vi "VISA02_ModbusRTU01_Read.vi"(11 "YTESTER测试数据":T1={"Socket(From1)"=1, "SN"=refnum, "StopFlagRef"=refnum, "YT System Queue"=refnum}) -> (3 "YTESTER结论":T2)   [LabVIEW 2017]
doc: "VIDescription=基于NI官方库的MODBUS操作"
uses:
  YtCommon.lvlibp/yt`Step StepBaseInput.ctl
  YtCommon.lvlibp/yt`Step StepResult.ctl
  YtCommon.lvlibp/yt`Step TestData.ctl
  YtCommon.lvlibp/yt`Step System Queue.ctl
  Step`s VIs/YYLLGeneric/variable_W.ctl
  YtCommon.lvlibp/yt`Data-Ytester Type Data.ctl
  Step`s VIs/NI Modbus.llb/MB Serial Master Query Read Discrete Inputs (poly).vi
  Step`s VIs/NI Modbus.llb/MB Serial Master Query Read Coils (poly).vi
  Step`s VIs/NI Modbus.llb/MB Serial Master Query Read Input Registers (poly).vi
  Step`s VIs/NI Modbus.llb/MB Serial Master Query Read Holding Registers (poly).vi
  YtCommon.lvlibp
panel:
  out "Read Registers":u16[](array[numeric]) format="%.0x"
  out "Read Bits":bool[](array[boolean])
  in  "YTESTER开放参数":T4={"YTESTER_BaseInput"={"isTest"=FALSE, "isSkip"=FALSE, "StepName"="NI Modbus读", "OnPass"=enum."Next", "OnFail"=enum."Next", "ReTestNumber"=0.0}, "VISA resource"="", "baud rate (9600)"="9600", "Mode"=enum."RTU", "ReadType"=enum."Discretes Input", "Slave Address"=1, "Timeout"=3000, "Starting Address"=0, "Quantity"=1} {"Starting Address" format="%.0x"}
  # "Modbus\nRead"
  # "#yyll 采用NI-Modbus VI 内部存在耗时，待优化！！！"
  # "Modbus四种数据类型：\n　　Discretes Input　　　　     位变量            只读\n　　Coils　　　　　　　　    　 位变量            读写\n　　Input Registers　　   　16-bit整型            只读\n　　Holding Registers 　    16-bit整型            读写"
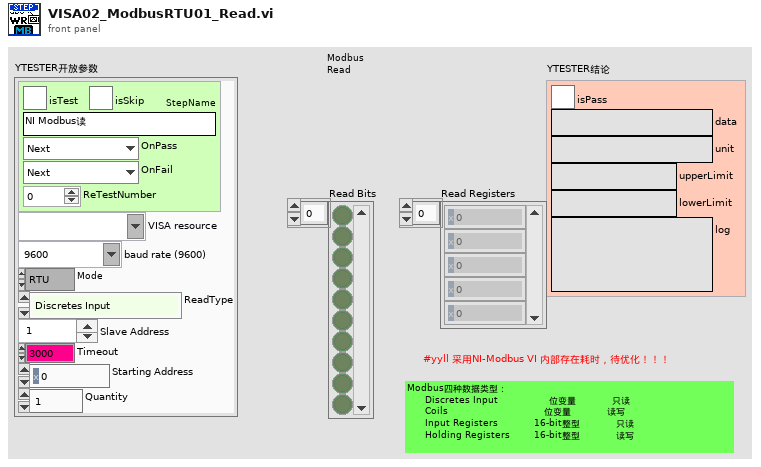
[diagram p1: front panel]
types:
  T1 = typedef "YtCommon.lvlibp/yt`Step TestData.ctl" = cluster{"Socket(From1)":i32, "SN":refnum<notifier>, "StopFlagRef":refnum<notifier>, "YT System Queue":refnum<queue>}
  T2 = typedef "YtCommon.lvlibp/yt`Step StepResult.ctl" = cluster{"isPass":bool, "data":string, "unit":string, "upperLimit":string, "lowerLimit":string, "log":string}
  T3 = typedef "YtCommon.lvlibp/yt`Step StepBaseInput.ctl" = cluster{"isTest":bool, "isSkip":bool, "StepName":string, "OnPass":enum16{"Next", "ToOVER", "Terminate"}, "OnFail":enum16{"Next", "ToOVER", "Terminate"}, "ReTestNumber":dbl}
  T4 = cluster{"YTESTER_BaseInput":T3, "VISA resource":refnum<visa-resource-name>, "baud rate (9600)":string, "Mode":enum16{"RTU", "ASCII"}, "ReadType":enum16{"Discretes Input", "Coils", "Input Registers", "Holding Registers"}, "Slave Address":u8, "Timeout":u32, "Starting Address":u16, "Quantity":u16}
  T5 = cluster{"Mode":enum16{"RTU", "ASCII"}, "Slave Address":u8}
  T6 = enum16{"Discretes Input", "Coils", "Input Registers", "Holding Registers"}
  T7 = typedef "variable_W.ctl" = cluster{"YT_TYPE":T8, "TypeData":string[], "Tips":string}
  T8 = typedef "YtCommon.lvlibp/yt`Data-Ytester Type Data.ctl" = enum16{"NULL", "NUM", "BOOL", "TXT", "ENUM", "TIME", "PATH", "VISA", "COMBO", "ColorBox", "RadioBtn", "Array_NUM", "Array_BOOL", "Array_TXT", "Array_ENUM", "Array_PATH", "Array_COMBO"}
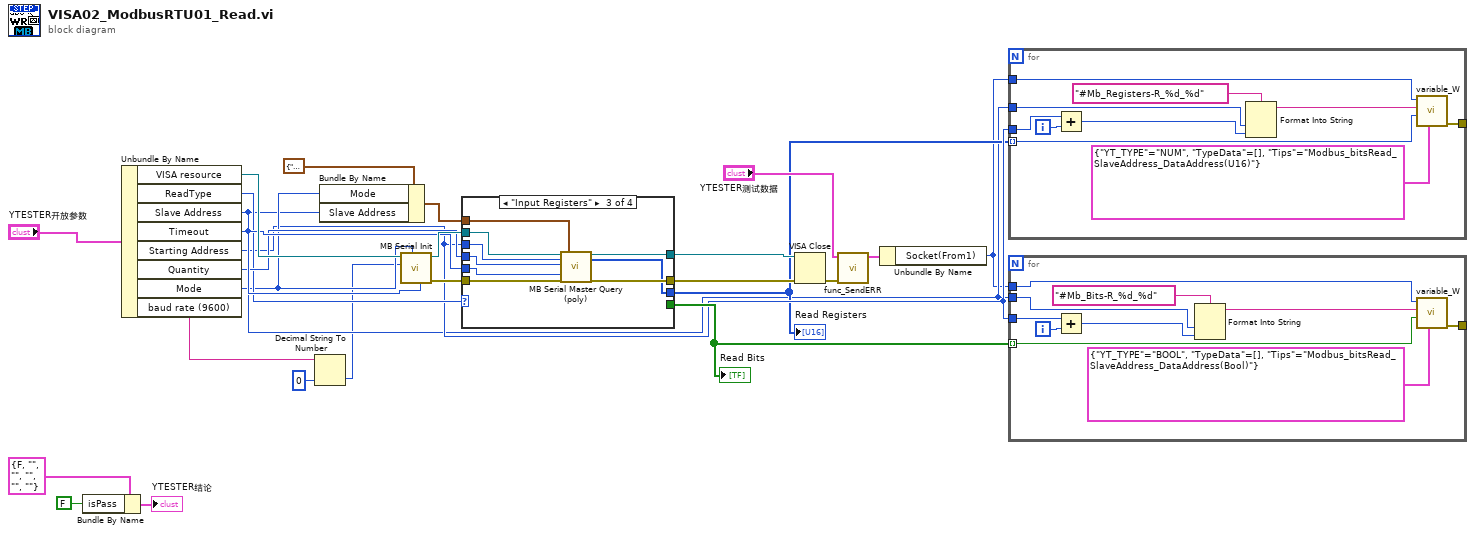
[diagram p0: block diagram]
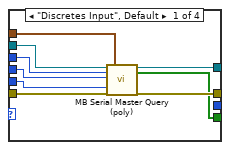
[diagram p2: hidden frame]
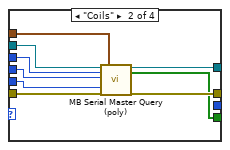
[diagram p3: hidden frame]
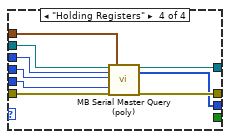
[diagram p4: hidden frame]
diagram:
  n1 = Bundle By Name(cluster=T2 {"isPass"=FALSE, "data"="", "unit"="", "upperLimit"="", "lowerLimit"="", "log"=""} ("Result"), "isPass"=FALSE) -> (→"YTESTER结论":T2)
  n2 = Unbundle By Name("YTESTER开放参数") -> ("VISA resource"=w18:refnum<visa-resource-name>, "ReadType"=w9:T6, "Slave Address"=w5:u8, "Timeout"=w15:u32, "Starting Address"=w7:u16, "Quantity"=w12:u16, "Mode"=w8:enum16{"RTU", "ASCII"}, "baud rate (9600)"=w2:string)
  n3 = Decimal String To Number(string=w2, default (0L)=u32 0 ("default (0 I32)")) -> (number=w1:u32)  [unwired: 1 in, 1 out]
  n4 = Bundle By Name(cluster=T5 {"Mode"=enum."RTU", "Slave Address"=0} ("Serial Parameters"), "Mode"=w8, "Slave Address"=w5) -> (w16:T5)
  n5 = call "MB Serial Init.vi"("Timeout"=w15, "Mode"=w8, "Baud Rate"=w1, "VISA resource name"=w18) -> ("error out"=w21:errorcluster, "VISA resource name out"=w23:refnum<visa-resource-name>)  [unwired: 3 in, 3 out]
  n6 = case shown="\"Input Registers\"" w9 {
    tunnel: w23 -> [w35 w44 w53 w62]
    tunnel: [w34 w43 w52 w61] -> w22
    tunnel: w21 -> [w33 w42 w51 w60]
    tunnel: [w32 w41 w50 w59] -> w20
    tunnel: w16 -> [w31 w40 w49 w58]
    tunnel: w15 -> [w30 w39 w48 w57]
    tunnel: w12 -> [w29 w38 w47 w56]
    tunnel: [w28 w37 _ _] -> w10
    tunnel: w7 -> [w27 w36 w46 w55]
    tunnel: [_ _ w45 w54] -> w6
    frame "Discretes Input", Default {
      n7 = call-poly "MB Serial Master Query (poly).vi"("VISA resource name"=w35, "Starting Address"=w27, "Quantity"=w29, "Timeout"=w30, "error in"=w33, "Serial Parameters"=w31) -> ("VISA resource name out"=w34:refnum<visa-resource-name>, "Discrete Inputs"=w28:bool[], "error out"=w32:errorcluster)  [unwired: 11 out]
    }
    frame "Coils" {
      n8 = call-poly "MB Serial Master Query (poly).vi"("VISA resource name"=w44, "Starting Address"=w36, "Quantity"=w38, "Timeout"=w39, "error in"=w42, "Serial Parameters"=w40) -> ("VISA resource name out"=w43:refnum<visa-resource-name>, "Coils"=w37:bool[], "error out"=w41:errorcluster)  [unwired: 11 out]
    }
    frame "Input Registers" {
      n9 = call-poly "MB Serial Master Query (poly).vi"("VISA resource name"=w53, "Starting Address"=w46, "Quantity"=w47, "Timeout"=w48, "error in"=w51, "Serial Parameters"=w49) -> ("VISA resource name out"=w52:refnum<visa-resource-name>, "Input Registers"=w45:u16[], "error out"=w50:errorcluster)  [unwired: 11 out]
    }
    frame "Holding Registers" {
      n10 = call-poly "MB Serial Master Query (poly).vi"("VISA resource name"=w62, "Starting Address"=w55, "Quantity"=w56, "Timeout"=w57, "error in"=w60, "Serial Parameters"=w58) -> ("VISA resource name out"=w61:refnum<visa-resource-name>, "Holding Registers"=w54:u16[], "error out"=w59:errorcluster)  [unwired: 11 out]
    }
  }
  "Read Bits" <- w10
  "Read Registers" <- w6
  n11 = VISA Close(VISA resource name=w22, error in (no error)=w20) -> (error out=w14:errorcluster)
  n12 = call "func_SendERR.vi"("ERR (String\\Errclust)"=w14, "YTESTER测试数据 in"="YTESTER测试数据") -> ("YTESTER测试数据 out"=w11:T1)  [unwired: 9 in]
  n13 = Unbundle By Name(w11) -> ("Socket(From1)"=w4:i32)
  n14 = for {
    tunnel: w4 -> [w72]
    tunnel: w6 -> [w71] mode=indexing
    tunnel: [w70] -> _
    tunnel: w5 -> [w66]
    tunnel: w7 -> [w65]
    i -> [w64]
    n15 = Add(x=w65, y=w64) -> (x+y=w63:i32)
    n16 = Format Into String(format string="#Mb_Registers-R_%d_%d", w66, w63) -> (resulting string=w67:string)  [unwired: 2 in, 1 out]
    n17 = call "variable_W.vi"("附加的Information"=T7 {"YT_TYPE"=enum."NUM", "TypeData"=[], "Tips"="Modbus_bitsRead_SlaveAddress_DataAddress(U16)"}, "待写入池的输入控件"=w71, "待写入池变量名称"=w67, "函数池名称 in"=w72) -> ("error out"=w70:errorcluster)  [unwired: 5 in, 2 out]
  }
  n18 = for {
    tunnel: w10 -> [w81] mode=indexing
    tunnel: [w80] -> _
    tunnel: w5 -> [w76]
    tunnel: w7 -> [w75]
    tunnel: w4 -> [w82]
    i -> [w74]
    n19 = Add(x=w75, y=w74) -> (x+y=w73:i32)
    n20 = Format Into String(format string="#Mb_Bits-R_%d_%d", w76, w73) -> (resulting string=w77:string)  [unwired: 2 in, 1 out]
    n21 = call "variable_W.vi"("附加的Information"=T7 {"YT_TYPE"=enum."BOOL", "TypeData"=[], "Tips"="Modbus_bitsRead_SlaveAddress_DataAddress(Bool)"}, "待写入池的输入控件"=w81, "待写入池变量名称"=w77, "函数池名称 in"=w82) -> ("error out"=w80:errorcluster)  [unwired: 5 in, 2 out]
  }
